vi "position test (SubVI).vi"(1 "Numeric":i32, 2 "String":string) -> (0 "Boolean":bool)   [LabVIEW 2013]
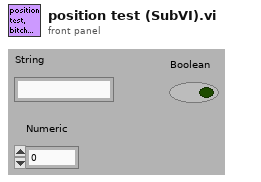
[diagram p1: front panel]
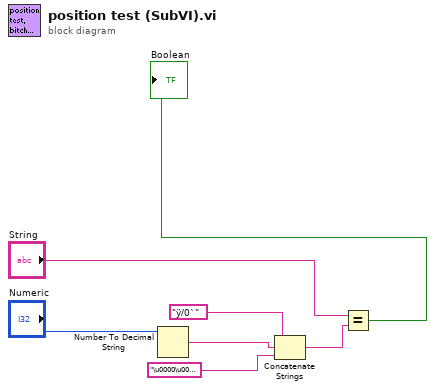
[diagram p0: block diagram]
diagram:
  n1 = Number To Decimal String(number="Numeric") -> (decimal integer string=w3:string)  [unwired: 1 in]
  n2 = Concatenate Strings("ÿ/0`" ("string"), w3, "\u0000\u0003\r\n" ("string")) -> (w4:string)
  n3 = Equal?(x="String", y=w4) -> (x = y?=→"Boolean":bool)
